vi "GObject Factory.vi"(7 "Owning VI":path, 10 "LangFile ref":refnum<data-value>, 11 "ClassName":string) -> (3 "GObject":refnum<class "GObject.lvclass">)   [LabVIEW 2013, in "SET Project Data.lvlib" / "VI Data.lvclass"]
uses:
  VI Data.lvclass
  Control Classes/GObject/GObject.lvclass
  Resource Data Class/Resource Data.lvclass
  Control Classes/Control/Control.lvclass
  Control Classes/BoolControl/BoolControl.lvclass
  Control Classes/RingControl/RingControl.lvclass
  Control Classes/TabControl/TabControl.lvclass
  Control Classes/ArrayControl/ArrayControl.lvclass
  Control Classes/StringControl/StringControl.lvclass
  Control Classes/WaveformChart/WaveformChart.lvclass
  Control Classes/IntensityChart/IntensityChart.lvclass
  Control Classes/IntensityGraph/IntensityGraph.lvclass
  Control Classes/GraphChart/GraphChart.lvclass
  Control Classes/WaveformGraph/WaveformGraph.lvclass
  Control Classes/DecorationText/DecorationText.lvclass
  Control Classes/StringConstant/StringConstant.lvclass
  Control Classes/ArrayConstant/ArrayConstant.lvclass
  Control Classes/FrontPanel/FrontPanel.lvclass
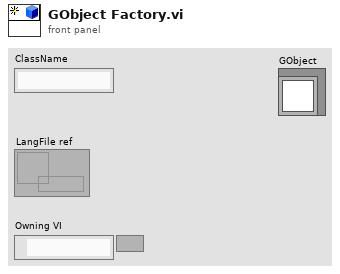
[diagram p1: front panel]
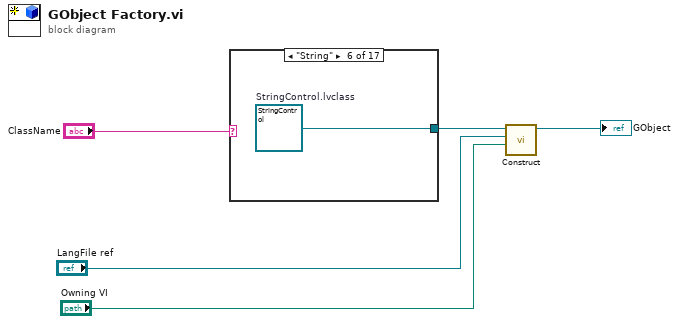
[diagram p0: block diagram]
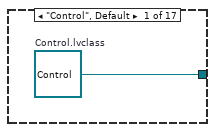
[diagram p2: hidden frame]
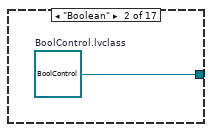
[diagram p3: hidden frame]
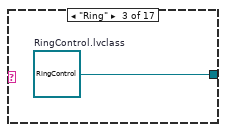
[diagram p4: hidden frame]
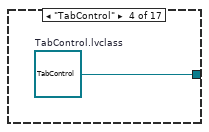
[diagram p5: hidden frame]
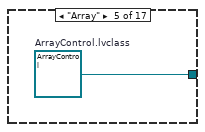
[diagram p6: hidden frame]
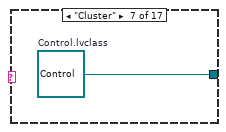
[diagram p7: hidden frame]
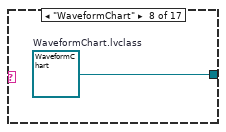
[diagram p8: hidden frame]
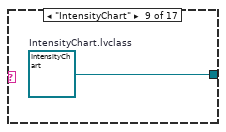
[diagram p9: hidden frame]
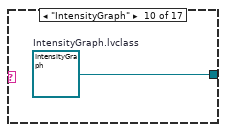
[diagram p10: hidden frame]
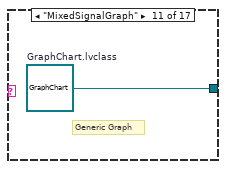
[diagram p11: hidden frame]
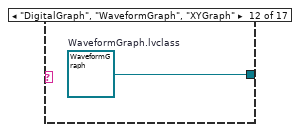
[diagram p12: hidden frame]
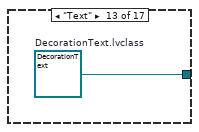
[diagram p13: hidden frame]
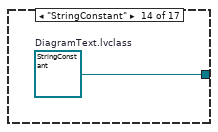
[diagram p14: hidden frame]
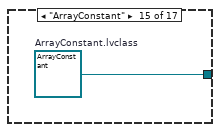
[diagram p15: hidden frame]
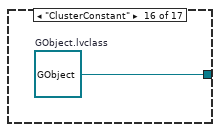
[diagram p16: hidden frame]
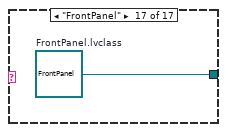
[diagram p17: hidden frame]
diagram:
  n1 = case shown="\"String\"" "ClassName" {
    tunnel: [w6 w7 w8 w9 w10 w11 w12 w13 w14 w15 w16 w17 w18 w19 w20 w21 w22] -> w4
    frame "Control", Default {
      w6 = refnum<class "Control.lvclass"> refnum  # Control.lvclass
    }
    frame "Boolean" {
      w7 = refnum<class "BoolControl.lvclass"> refnum  # BoolControl.lvclass
    }
    frame "Ring" {
      w8 = refnum<class "RingControl.lvclass"> refnum  # RingControl.lvclass
    }
    frame "TabControl" {
      w9 = refnum<class "TabControl.lvclass"> refnum  # TabControl.lvclass
    }
    frame "Array" {
      w10 = refnum<class "ArrayControl.lvclass"> refnum  # ArrayControl.lvclass
    }
    frame "String" {
      w11 = refnum<class "StringControl.lvclass"> refnum  # StringControl.lvclass
    }
    frame "Cluster" {
      w12 = refnum<class "Control.lvclass"> refnum  # Control.lvclass
    }
    frame "WaveformChart" {
      w13 = refnum<class "WaveformChart.lvclass"> refnum  # WaveformChart.lvclass
    }
    frame "IntensityChart" {
      w14 = refnum<class "IntensityChart.lvclass"> refnum  # IntensityChart.lvclass
    }
    frame "IntensityGraph" {
      w15 = refnum<class "IntensityGraph.lvclass"> refnum  # IntensityGraph.lvclass
    }
    frame "MixedSignalGraph" {
      w16 = refnum<class "GraphChart.lvclass"> refnum  # GraphChart.lvclass
      # "Generic Graph"
    }
    frame "DigitalGraph", "WaveformGraph", "XYGraph" {
      w17 = refnum<class "WaveformGraph.lvclass"> refnum  # WaveformGraph.lvclass
    }
    frame "Text" {
      w18 = refnum<class "DecorationText.lvclass"> refnum  # DecorationText.lvclass
    }
    frame "StringConstant" {
      w19 = refnum<class "StringConstant.lvclass"> refnum  # DiagramText.lvclass
    }
    frame "ArrayConstant" {
      w20 = refnum<class "ArrayConstant.lvclass"> refnum  # ArrayConstant.lvclass
    }
    frame "ClusterConstant" {
      w21 = refnum<class "GObject.lvclass"> refnum  # GObject.lvclass
    }
    frame "FrontPanel" {
      w22 = refnum<class "FrontPanel.lvclass"> refnum  # FrontPanel.lvclass
    }
  }
  n2 = call "Construct.vi"("Owning VI"="Owning VI", "LangFile ref"="LangFile ref", "GObject in"=w4) -> ("GObject out"=→"GObject":refnum<class "GObject.lvclass">)  [unwired: 7 in, 1 out]
